vi "StahlPS_USB.destructor.vi"(0 "i ref in":refnum<vi>, 5 "error in(no error)":errorcluster) -> (19 "error out":errorcluster)   [LabVIEW 2014, in "StahlPS_USB.lvlib"]
doc: "This is the destructor of a class.\n\nLicense Agreement for this software:\n\nCopyright (C)\nGesellschaft für Schwerionenforschung, GSI\nPlanckstr. 1\n64291 Darmstadt\nGermany\n\nContact: D.Beck@gsi.de \n\nThis program is free software; you can redistribute it and/or modify it under the terms of the \nGNU General Public License as published by the Free Software Foundation; either version 2 of \nthe license, or (at your option) any later version.\n\nThis program is distributed in the hope that it will be useful, but WITHOUT ANY WARRANTY; \nwithout even the implied warranty of MERCHANTABILITY or FITNESS FOR A PARTICULAR PURPOSE. See the GNU General License for more details (http://www.gnu.org).\n\nGesellschaft für Schwerionenforschung, GSI\nPlanckstr. 1, 64291 Darmstadt, Germany\nFor all questions and ideas contact: M.Richter@gsi.de, H.Brand@gsi.de or D.Beck@gsi.de.\nLast update: 16-JUN-2004"
uses:
  StahlPS_USB.lvlib
  CSCore/CSApplicationBaseClasses/PSChannelBase/PSChannelBase.lvlib
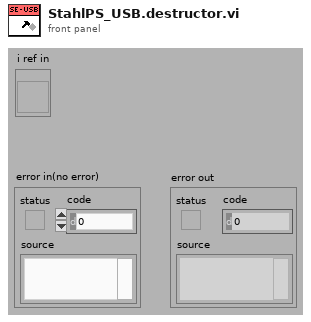
[diagram p1: front panel]
types:
  T1 = typedef "StahlPS_USB.lvlib/StahlPS_USB.i attribute.ctl" = cluster{"VISA resource name":refnum<visa-resource-name>, "Type":string, "MaxVoltage":dbl, "MinVoltage":dbl, "Elektrode Names":string[]}
  T2 = enum16{"SetAttribute", "GetAttribute", "CreateAttribute", "DestroyAttribute", "DestroyAllAtributes"}
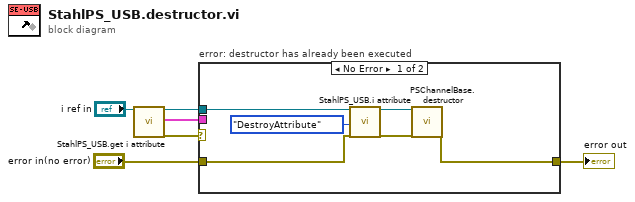
[diagram p0: block diagram]
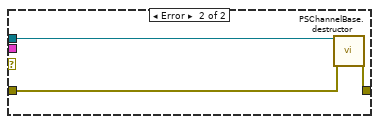
[diagram p2: hidden frame]
diagram:
  n1 = call "StahlPS_USB.get i attribute.vi"("i ref in"="i ref in") -> ("i ref out"=w5:refnum<vi>, "i attribute"=w4:T1, "error out"=w3:errorcluster)  [unwired: 16 in]
  n2 = case "error: destructor has already been executed" shown="No Error" w3 {
    tunnel: [w9 w13] -> w1
    tunnel: "error in(no error)" -> [w7 w14]
    tunnel: w5 -> [w8 w15]
    tunnel: w4 -> [_ _]
    frame No Error {
      n3 = call "StahlPS_USB.i attribute.vi"("VI Refnum"=w8, "Action"=T2."DestroyAttribute", "error in (no error)"=w7) -> ("VI Refnum out"=w11:refnum<vi>, "error out"=w10:errorcluster)  [unwired: 14 in, 1 out]
      n4 = call "PSChannelBase.destructor.vi"("i ref in"=w11, "error in (no error)"=w10) -> ("error out"=w9:errorcluster)  [unwired: 17 in]
    }
    frame Error {
      n5 = call "PSChannelBase.destructor.vi"("i ref in"=w15, "error in (no error)"=w14) -> ("error out"=w13:errorcluster)  [unwired: 17 in]
    }
  }
  "error out" <- w1
